vi "FTW-CodeGen-GetTerms.vi"(0 "State In":T2, 5 "XRef":refnum<vi>) -> (4 "Terms":T1(array[cluster]))   [LabVIEW 2015, in "FTW-Dataflow-Synchronizer.xnode"]
uses:
  FTW-Dataflow-Synchronizer.xnode
  FTW-CodeGen-State.ctl
panel:
  # "Inputs"
  # "Outputs"
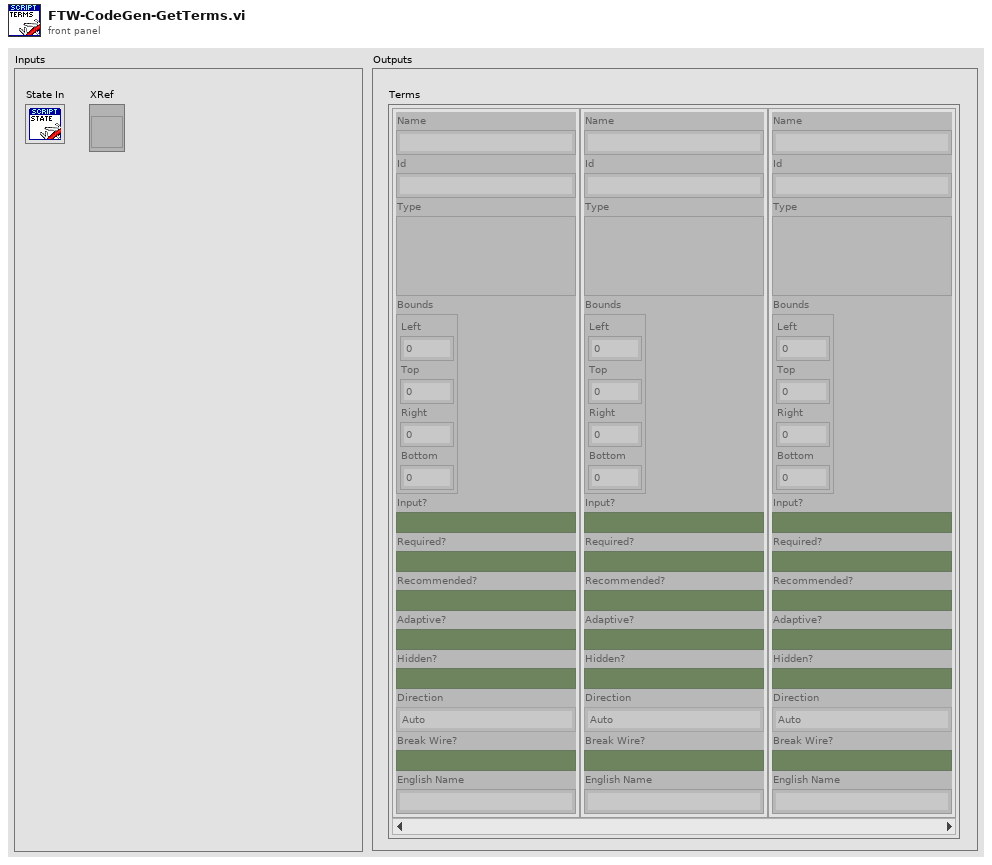
[diagram p1: front panel]
types:
  T1 = cluster{"Name":string, "Id":string, "Type":variant, "Bounds":cluster{"Left":i32, "Top":i32, "Right":i32, "Bottom":i32}, "Input?":bool, "Required?":bool, "Recommended?":bool, "Adaptive?":bool, "Hidden?":bool, "Direction":enum32{"Auto", "Up", "Down", "Left", "Right", "Center"}, "Break Wire?":bool, "English Name":string}[]
  T2 = typedef "FTW-Dataflow-Synchronizer.xnode/FTW-CodeGen-State.ctl" = cluster{"InputTerminals":cluster{"Wired?":bool, "ID":string, "DataName":string, "DataColor":u32, "Type":variant}[], "EnableTiming?":bool}
  T3 = cluster{"Wired?":bool, "ID":string, "DataName":string, "DataColor":u32, "Type":variant}[]
  T4 = enum32{"Auto", "Up", "Down", "Left", "Right", "Center"}
  T5 = cluster{"Name":string, "ID":string, "Type":variant, "Bounds":cluster{"Left":i32, "Top":i32, "Right":i32, "Bottom":i32}, "Input?":bool, "Required?":bool, "Recommended?":bool, "Adaptive?":bool, "Hidden?":bool, "Direction":enum32{"Auto", "Up", "Down", "Left", "Right", "Center"}, "Break Wire?":bool, "English Name":string}
  T6 = cluster{"Name":string, "ID":string, "Type":variant, "Bounds":cluster{"Left":i32, "Top":i32, "Right":i32, "Bottom":i32}, "Input?":bool, "Required?":bool, "Recommended?":bool, "Adaptive?":bool, "Hidden?":bool, "Direction":enum32{"Auto", "Up", "Down", "Left", "Right", "Center"}, "Break Wire?":bool, "English Name":string}[]
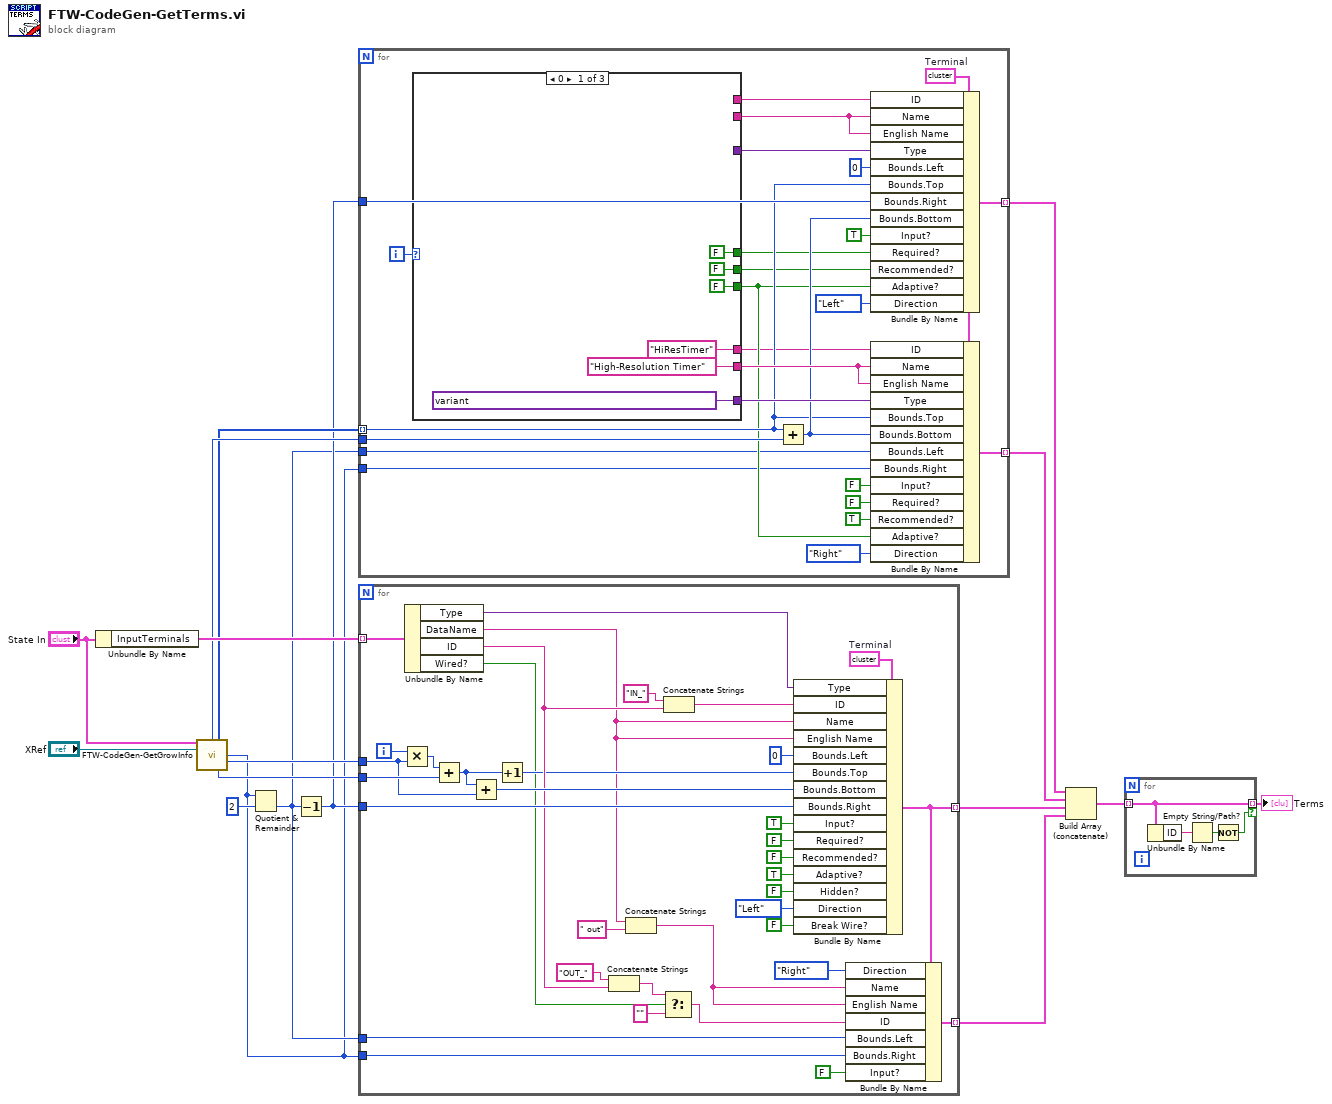
[diagram p0: block diagram]
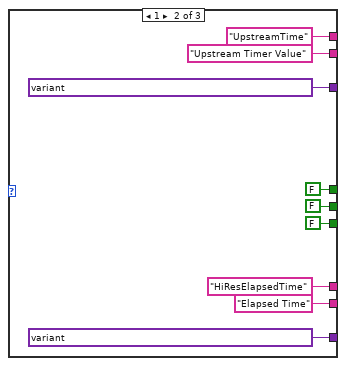
[diagram p2: hidden frame]
diagram:
  n1 = Unbundle By Name("State In") -> ("InputTerminals"=w13:T3)
  n2 = call "FTW-CodeGen-GetGrowInfo.vi"("State In"="State In", "XRef"="XRef") -> ("Timing Terminal Height"=w8:i32, "Timing Terminals"=w7:i32[], "Width"=w2:i32, "Terminal Height"=w9:i32, "Total Top Banner Height"=w14:i32)  [unwired: 5 in, 4 out]
  n3 = Quotient & Remainder(x=w2, y=2) -> (floor(x/y)=w3:i32)  [unwired: 1 out]
  n4 = Decrement(x=w3) -> (x-1=w4:i32)
  n5 = for {
    tunnel: [w42] -> w10 mode=indexing
    tunnel: w8 -> [w33]
    tunnel: w7 -> [w27] mode=indexing
    tunnel: [w38] -> w6 mode=indexing
    tunnel: w4 -> [w34]
    tunnel: w3 -> [w21]
    tunnel: w2 -> [w22]
    i -> [w25]
    w18 = T5 {"Name"="", "ID"="", "Type"=variant, "Bounds"={"Left"=0, "Top"=0, "Right"=0, "Bottom"=0}, "Input?"=FALSE, "Required?"=FALSE, "Recommended?"=FALSE, "Adaptive?"=FALSE, "Hidden?"=FALSE, "Direction"=enum."Auto", "Break Wire?"=FALSE, "English Name"=""}  # Terminal
    n6 = case shown="0" w25 {
      tunnel: [_ "Upstream Timer Value" ("Name") _] -> w43
      tunnel: [_ variant(dbl 0.0) ("variant") _] -> w41
      tunnel: ["High-Resolution Timer" ("Name") "Elapsed Time" ("Name") _] -> w35
      tunnel: [variant(dbl 0.0) ("variant") variant(dbl 0.0) ("variant") _] -> w36
      tunnel: [FALSE ("Required?") FALSE ("Required?") _] -> w24
      tunnel: [FALSE ("Recommended?") FALSE ("Recommended?") _] -> w23
      tunnel: [FALSE ("Adaptive?") FALSE ("Adaptive?") _] -> w26
      tunnel: [_ "UpstreamTime" ("ID") _] -> w19
      tunnel: ["HiResTimer" ("ID") "HiResElapsedTime" ("ID") _] -> w20
      frame 0 {
      }
      frame 1 {
      }
      frame Default {
      }
    }
    n7 = Add(x=w27, y=w33) -> (x+y=w32:i32)
    n8 = Bundle By Name(cluster=w18, "ID"=w19, "Name"=w43, "English Name"=w43, "Type"=w41, "Bounds.Left"=0, "Bounds.Top"=w27, "Bounds.Right"=w34, "Bounds.Bottom"=w32, "Input?"=TRUE, "Required?"=w24, "Recommended?"=w23, "Adaptive?"=w26, "Direction"=T4."Left") -> (w42:T5)
    n9 = Bundle By Name(cluster=w18, "ID"=w20, "Name"=w35, "English Name"=w35, "Type"=w36, "Bounds.Top"=w27, "Bounds.Bottom"=w32, "Bounds.Left"=w21, "Bounds.Right"=w22, "Input?"=FALSE, "Required?"=FALSE, "Recommended?"=TRUE, "Adaptive?"=w26, "Direction"=T4."Right") -> (w38:T5)
  }
  n10 = for {
    tunnel: w9 -> [w85]
    tunnel: w14 -> [w86]
    tunnel: w4 -> [w82]
    tunnel: w2 -> [w83]
    tunnel: w3 -> [w84]
    tunnel: w13 -> [w79] mode=indexing
    tunnel: [w76] -> w12 mode=indexing
    tunnel: [w75] -> w11 mode=indexing
    i -> [w78]
    w69 = T5 {"Name"="", "ID"="", "Type"=variant, "Bounds"={"Left"=0, "Top"=0, "Right"=0, "Bottom"=0}, "Input?"=FALSE, "Required?"=FALSE, "Recommended?"=FALSE, "Adaptive?"=FALSE, "Hidden?"=FALSE, "Direction"=enum."Auto", "Break Wire?"=FALSE, "English Name"=""}  # Terminal
    n11 = Multiply(x=w78, y=w85) -> (x*y=w87:i32)
    n12 = Unbundle By Name(w79) -> ("Type"=w63:variant, "DataName"=w62:string, "ID"=w70:string, "Wired?"=w61:bool)
    n13 = Add(x=w87, y=w86) -> (x+y=w81:i32)
    n14 = Add(x=w81, y=w85) -> (x+y=w80:i32)
    n15 = Increment(x=w81) -> (x+1=w64:i32)
    n16 = Concatenate Strings("OUT_" ("format string"), w70) -> (w67:string)
    n17 = Concatenate Strings(w62, " out" ("string")) -> (w65:string)
    n18 = Select(t=w67, s=w61, f="") -> (s? t:f=w59:string)
    n19 = Concatenate Strings("IN_" ("format string"), w70) -> (w60:string)
    n20 = Bundle By Name(cluster=w69, "Type"=w63, "ID"=w60, "Name"=w62, "English Name"=w62, "Bounds.Left"=0, "Bounds.Top"=w64, "Bounds.Bottom"=w80, "Bounds.Right"=w82, "Input?"=TRUE, "Required?"=FALSE, "Recommended?"=FALSE, "Adaptive?"=TRUE, "Hidden?"=FALSE, "Direction"=T4."Left", "Break Wire?"=FALSE) -> (w76:T5)
    n21 = Bundle By Name(cluster=w76, "Direction"=T4."Right", "Name"=w65, "English Name"=w65, "ID"=w59, "Bounds.Left"=w84, "Bounds.Right"=w83, "Input?"=FALSE) -> (w75:T5)
  }
  n22 = Build Array (concatenate)(w10, w6, w12, w11) -> (w1:T6)
  n23 = for {
    tunnel: w1 -> [w98] mode=indexing
    tunnel: [w98] -> w5 mode=indexing if=w95
    n24 = Unbundle By Name(w98) -> ("ID"=w96:string)
    n25 = Empty String/Path?(string/path=w96) -> (empty?=w97:bool)
    n26 = Not(x=w97) -> (.not. x?=w95:bool)
  }
  "Terms" <- w5
